vi "ODFT_iHV.vi"(10 "Ext_HV":dbl=38.0 format="%#_13g", 11 "Semiconductor Module Context":T1) -> (0 "error out":errorcluster)   [LabVIEW 2013]
uses:
  <vilib>/NI_TestStand_SemiconductorModule/NI_TestStand_Semiconductor_Module.lvlibp/PinMap/General/SemiconductorModuleContext.ctl
  <instrlib>/niHSDIO/niHSDIO.llb/niHSDIO_ctl Trigger Script - trigID Values (Ring).ctl
  <vilib>/NI_TestStand_SemiconductorModule/NI_TestStand_Semiconductor_Module.lvlibp/PinMap/DC Power/PinsToNIDCPowerSessions.vi
  <vilib>/NI_TestStand_SemiconductorModule/NI_TestStand_Semiconductor_Module.lvlibp/PinMap/Deprecated/PublishDataDoubleMultiplePinsMultipleInstruments.vi
  <vilib>/NI_TestStand_SemiconductorModule/NI_TestStand_Semiconductor_Module.lvlibp
panel:
  out "current measurements":dbl[][][](array[numeric])
  in  "Pins":string[](array[string])=["HV"]
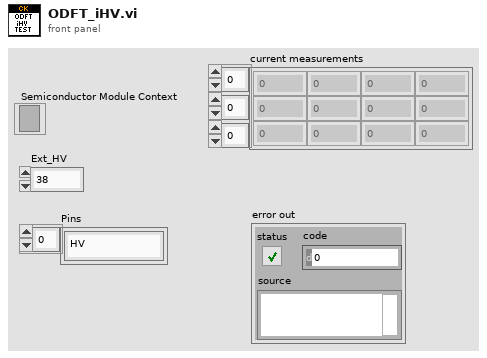
[diagram p1: front panel]
types:
  T1 = typedef "NI_TestStand_Semiconductor_Module.lvlibp/SemiconductorModuleContext.ctl" = refnum<k7>
  T2 = typedef "niHSDIO_ctl Trigger Script - trigID Values (Ring).ctl" = string
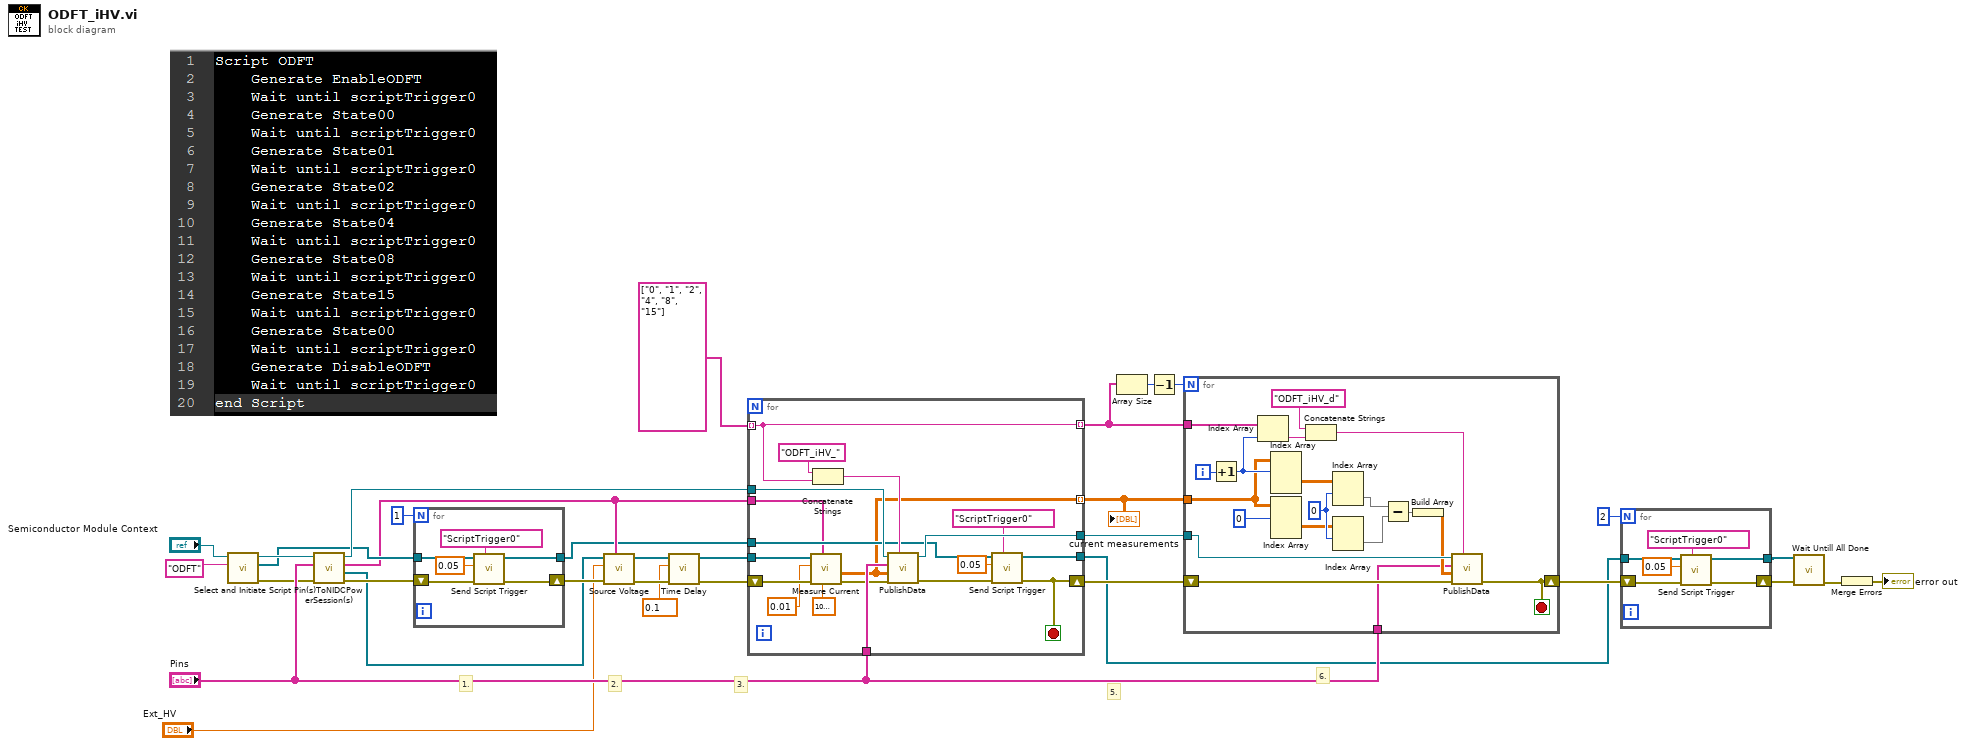
[diagram p0: block diagram]
diagram:
  # "3."
  # "6."
  # "5."
  # "2."
  # "1."
  n1 = call "Select and Initiate Script.vi"("script name"="ODFT", "Semiconductor Module Context"="Semiconductor Module Context") -> ("error out"=w15:errorcluster, "HSDIO GEN Sessions Out"=w16:refnum<k15>[], "Semiconductor Module Context Out"=w17:T1)  [unwired: 7 in]
  n2 = call-poly <vilib>:"Pin(s)ToNIDCPowerSession(s).vi"("error in (no error)"=w15, "Pins"="Pins", "Semiconductor Module Context"=w17) -> ("error out"=w31:errorcluster, "Instrument Sessions"=w14:refnum<k15>[], "Channel Lists"=w13:string[], "Semiconductor Module Context Out"=w19:T1)  [unwired: 4 in, 1 out]
  n3 = for {
    N: 1 -> [_]
    shift-right: [w36] -> w29
    shift-left: w31 -> [w37]
    tunnel: w16 -> [w35]
    tunnel: [w34] -> w11
    n4 = call "Send Script Trigger.vi"("trigger id (script trigger 0)"=T2 "ScriptTrigger0", "error in (no error)"=w37, "Delay Time (s)"=0.05, "HSDIO Sessions In"=w35) -> ("error out"=w36:errorcluster, "HSDIO Sessions Out"=w34:refnum<k15>[])  [unwired: 6 in]
  }
  n5 = call "Source Voltage.vi"("Channel Lists"=w13, "error in (no error)"=w29, "voltage level"="Ext_HV", "Instrument Sessions In"=w14) -> ("error out"=w9:errorcluster, "Instrument Sessions Out"=w28:refnum<k15>[])  [unwired: 4 in, 2 out]
  n6 = call "Time Delay"("error in (no error)"=w9, "Delay Time (s)"=0.1) -> ("error out"=w8:errorcluster)  [unwired: 9 in]
  n7 = for {
    tunnel: string[] ["0", "1", "2", "4", "8", "15"] -> [w54] mode=indexing
    tunnel: w28 -> [w44]
    tunnel: w19 -> [w55]
    shift-right: [w48] -> w26
    shift-left: w8 -> [w46]
    tunnel: [w54] -> w24 mode=indexing
    tunnel: "Pins" -> [w53]
    tunnel: w11 -> [w49]
    tunnel: [w52] -> w21
    tunnel: w13 -> [w43]
    tunnel: [w47] -> w10 mode=indexing
    tunnel: [w40] -> w4
    stop <- w48 stop-if-true
    n8 = call "Measure Current.vi"("Result Multiplier"=1000000.0, "Channel Lists"=w43, "error in (no error)"=w46, "Delay Time (s)"=0.01, "DCPower Sessions In"=w44) -> ("error out"=w45:errorcluster, "current measurements"=w47:dbl[][])  [unwired: 4 in, 1 out]
    n9 = Concatenate Strings("ODFT_iHV_", w54) -> (w57:string)
    n10 = call-poly <vilib>:"PublishData.vi"("Measurement Id"=w57, "error in (no error)"=w45, "Data In"=w47, "Pins"=w53, "Semiconductor Module Context"=w55) -> ("error out"=w51:errorcluster, "Semiconductor Module Context Out"=w52:T1)  [unwired: 5 in]
    n11 = call "Send Script Trigger.vi"("trigger id (script trigger 0)"=T2 "ScriptTrigger0", "error in (no error)"=w51, "Delay Time (s)"=0.05, "HSDIO Sessions In"=w49) -> ("error out"=w48:errorcluster, "HSDIO Sessions Out"=w40:refnum<k15>[])  [unwired: 6 in]
  }
  "current measurements" <- w10
  n12 = Array Size(array=w24) -> (size(s)=w23:i32)
  n13 = Decrement(x=w23) -> (x-1=w22:i32)
  n14 = for {
    N: w22 -> [_]
    tunnel: w24 -> [w73]
    shift-right: [w66] -> w5
    shift-left: w26 -> [w71]
    tunnel: "Pins" -> [w58]
    tunnel: w21 -> [w67]
    tunnel: w10 -> [w65]
    i -> [w74]
    stop <- w66 stop-if-true
    w68 = 0 ("index (page)")
    n15 = Increment(x=w74) -> (x+1=w69:i32)
    n16 = Index Array(array=w73, index=w69) -> (element=w72:string)
    n17 = Index Array(array=w65, index (dim 0)=w69) -> (element=w64:dbl[][])  [unwired: 2 in]
    n18 = Index Array(array=w65, index (dim 0)=0 ("index (page)")) -> (element=w63:dbl[][])  [unwired: 2 in]
    n19 = Concatenate Strings("ODFT_iHV_d", w72) -> (w75:string)
    n20 = Index Array(array=w64, index (row)=w68) -> (element=w61:dbl[])  [unwired: 1 in]
    n21 = Index Array(array=w63, index (row)=w68) -> (element=w62:dbl[])  [unwired: 1 in]
    n22 = Subtract(x=w61, y=w62) -> (x-y=w60:dbl[])
    n23 = Build Array(w60) -> (w59:dbl[][])
    n24 = call-poly <vilib>:"PublishData.vi"("Measurement Id"=w75, "error in (no error)"=w71, "Data In"=w59, "Pins"=w58, "Semiconductor Module Context"=w67) -> ("error out"=w66:errorcluster)  [unwired: 5 in, 1 out]
  }
  n25 = for {
    N: 2 -> [_]
    shift-right: [w80] -> w2
    shift-left: w5 -> [w81]
    tunnel: w4 -> [w79]
    tunnel: [w78] -> w3
    n26 = call "Send Script Trigger.vi"("trigger id (script trigger 0)"=T2 "ScriptTrigger0", "error in (no error)"=w81, "Delay Time (s)"=0.05, "HSDIO Sessions In"=w79) -> ("error out"=w80:errorcluster, "HSDIO Sessions Out"=w78:refnum<k15>[])  [unwired: 6 in]
  }
  n27 = call "Wait Untill All Done.vi"("error in (no error)"=w2, "HSDIO Sessions In"=w3) -> ("error out"=w12:errorcluster)  [unwired: 8 in, 1 out]
  n28 = Merge Errors(w12) -> (→"error out":errorcluster)
